vi "Flatten and Set String Property.vi"(8 "error in (no error)":errorcluster, 9 "Value":variant, 10 "Property Name":string, 11 "Section Ref in":T1 format="%.0x") -> (0 "error out":errorcluster, 3 "Section Ref out":T1 format="%.0x")   [LabVIEW 2015, in "DCM Shared.lvlib"]
uses:
  DCM Shared.lvlib
  <vilib>/NI Veristand/Custom Device API/Custom Device Item Ref.ctl
  <vilib>/NI Veristand/Custom Device API/Set Item Property (String).vi
  <vilib>/NI VeriStand/Custom Device API/Custom Device API.lvlib
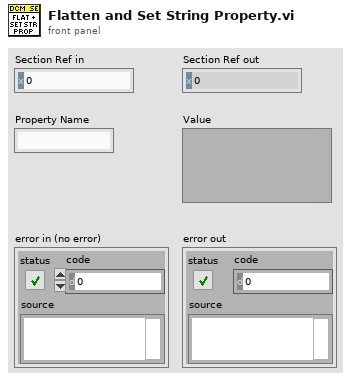
[diagram p1: front panel]
types:
  T1 = typedef "Custom Device API.lvlib/Custom Device Item Ref.ctl" = u64
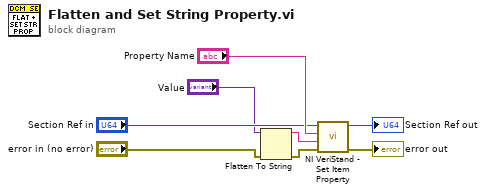
[diagram p0: block diagram]
diagram:
  n1 = Flatten To String(anything="Value", error in (no error)="error in (no error)") -> (data string=w8:string, error out=w2:errorcluster)  [unwired: 2 in, 1 out]
  n2 = call-poly <vilib>:"NI VeriStand - Set Item Property.vi"("error in (no error)"=w2, "Value"=w8, "Property Name"="Property Name", "Item Ref in"="Section Ref in") -> ("error out"=→"error out":errorcluster, "Item Ref out"=→"Section Ref out":T1)  [unwired: 5 in, 1 out]
